vi "FGVExcitationParameters.vi"(6 "Excitation In":T1={"Excitation"={"Frequency"=0.0, "Amplitude"=0.0, "DC Offset"=0.0, "Cut Off"=0.0, "RaPF"=FALSE, "Shift"=0.0}, "Background"={"Lift Height"=0.0, "Average Count"=12}, "Signal"=0} {"Signal" items=["Sine Wave", "Triangle Wave", "Square Wave", "Sawtooth Wave"]; "Background"."Average Count" items=["1", "2", "4", "8", "16", "32", "64", "128", "256", "512", "1024", "2048", "4096", "8192", "16384"]; "Background"."Lift Height" format="%.0pm"; "Excitation"."Shift" min=-100.0 max=100.0 format="%_1p%"; "Excitation"."Cut Off" format="%.0p%"; "Excitation"."DC Offset" format="%.0pm"; "Excitation"."Amplitude" format="%.0pm"; "Excitation"."Frequency" format="%.0pHz"}, 7 "Enum":T4, 8 "error in":errorcluster, 9 "lineFitThreshold In":dbl, 10 "syncParameters In":T3, 11 "Sensitivities In":T2={"inputSensitivity"=0.001506, "outputSensitivity"=664.01}) -> (0 "error out":errorcluster, 1 "lineFitThreshold Out":dbl, 2 "syncParameters Out":T3, 3 "Sensitivities Out":T2, 4 "Excitation Out":T1={"Excitation"={"Frequency"=0.0, "Amplitude"=0.0, "DC Offset"=0.0, "Cut Off"=0.0, "RaPF"=FALSE, "Shift"=0.0}, "Background"={"Lift Height"=0.0, "Average Count"=12}, "Signal"=0} {"Signal" items=["Sine Wave", "Triangle Wave", "Square Wave", "Sawtooth Wave"]; "Background"."Average Count" items=["1", "2", "4", "8", "16", "32", "64", "128", "256", "512", "1024", "2048", "4096", "8192", "16384"]; "Background"."Lift Height" format="%.0pm"; "Excitation"."Shift" min=-100.0 max=100.0 format="%_1p%"; "Excitation"."Cut Off" format="%.0p%"; "Excitation"."DC Offset" format="%.0pm"; "Excitation"."Amplitude" format="%.0pm"; "Excitation"."Frequency" format="%.0pHz"})   [LabVIEW 2016]
uses:
  controls/Enum.ctl
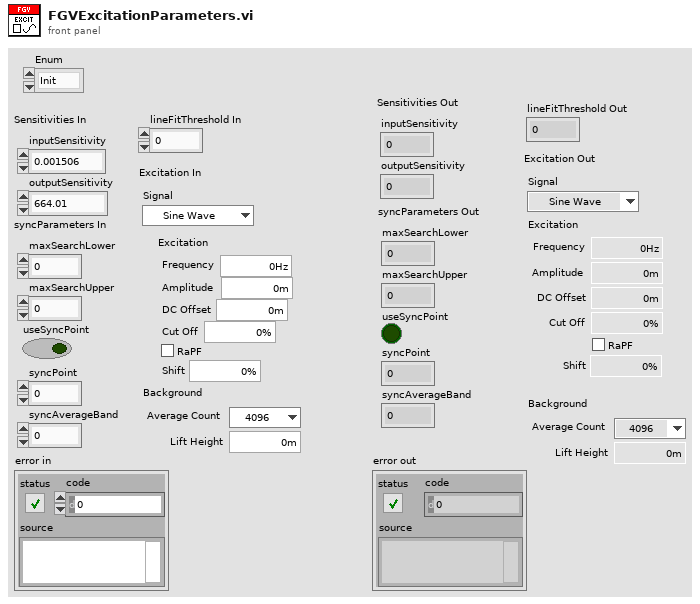
[diagram p1: front panel]
types:
  T1 = cluster{"Excitation":cluster{"Frequency":dbl, "Amplitude":dbl, "DC Offset":dbl, "Cut Off":dbl, "RaPF":bool, "Shift":dbl}, "Background":cluster{"Lift Height":dbl, "Average Count":u16}, "Signal":u16}
  T2 = cluster{"inputSensitivity":dbl, "outputSensitivity":dbl}
  T3 = cluster{"maxSearchLower":u16, "maxSearchUpper":u16, "useSyncPoint":bool, "syncPoint":u16, "syncAverageBand":u16}
  T4 = typedef "Enum.ctl" = enum16{"Init", "Read", "Write"}
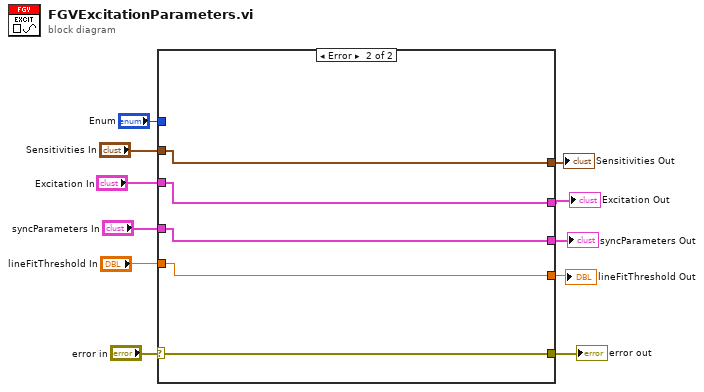
[diagram p0: block diagram]
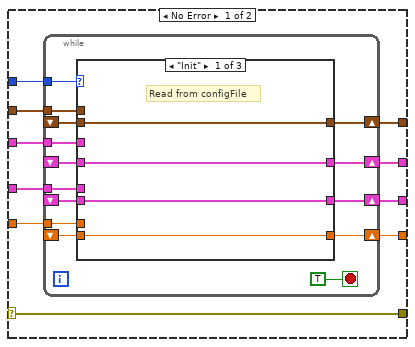
[diagram p2: hidden frame]
diagram:
  n1 = case shown="Error" "error in" {
    selector: "error in" -> [w20 w52]
    tunnel: "Enum" -> [w21 _]
    tunnel: [w20 w52] -> w10
    tunnel: "lineFitThreshold In" -> [w19 w51]
    tunnel: [w18 w51] -> w3
    tunnel: "Sensitivities In" -> [w16 w50]
    tunnel: [w17 w50] -> w5
    tunnel: "syncParameters In" -> [w15 w49]
    tunnel: [w14 w49] -> w6
    tunnel: "Excitation In" -> [w13 w48]
    tunnel: [w12 w48] -> w1
    frame No Error {
      n2 = while {
        tunnel: w21 -> [w34]
        tunnel: w19 -> [w33]
        shift-right: [w32] -> w18
        shift-left: _ -> [w31]
        tunnel: w16 -> [w28]
        shift-right: [w29] -> w17
        shift-left: _ -> [w30]
        tunnel: w15 -> [w27]
        shift-right: [w26] -> w14
        shift-left: _ -> [w25]
        tunnel: w13 -> [w24]
        shift-right: [w23] -> w12
        shift-left: _ -> [w22]
        stop <- TRUE stop-if-true
        n3 = case shown="\"Init\"" w34 {
          tunnel: w33 -> [_ _ w47]
          tunnel: [w39 w43 w47] -> w32
          tunnel: w31 -> [w39 w43 _]
          tunnel: w28 -> [_ _ w46]
          tunnel: [w38 w42 w46] -> w29
          tunnel: w30 -> [w38 w42 _]
          tunnel: w27 -> [_ _ w45]
          tunnel: [w37 w41 w45] -> w26
          tunnel: w25 -> [w37 w41 _]
          tunnel: w24 -> [_ _ w44]
          tunnel: [w36 w40 w44] -> w23
          tunnel: w22 -> [w36 w40 _]
          frame "Init" {
            # "Read from configFile"
          }
          frame "Read", Default {
          }
          frame "Write" {
          }
        }
      }
    }
    frame Error {
    }
  }
  "error out" <- w10
  "syncParameters Out" <- w6
  "Sensitivities Out" <- w5
  "Excitation Out" <- w1
  "lineFitThreshold Out" <- w3
